vi "getObjectPrivateData.vi"(8 "error in (no error)":errorcluster, 10 "object in":refnum<class>) -> (0 "error out":errorcluster, 3 "private data":variant[](array[variant]), 5 "interitance classes":string[](array[string]), 7 "versions":T1(array[cluster]))   [LabVIEW 2020, in "JKI JSON Object Serialization.lvlib" / "OOP_Utility.lvlib" / "Reflection.lvclass"]
doc: "This VI returns the class names, and private data values for the class hierarchy (top to bottom) of the input object. \n\nGCraftsman JSON Object Serialization Toolkit\nwww.GCraftsman.com\nCopyright (c) 2017, GCraftsman"
uses:
  Reflection.lvclass
  reflectionPoolAction.ctl
  Reflection.lvclass/Reflection.ctl
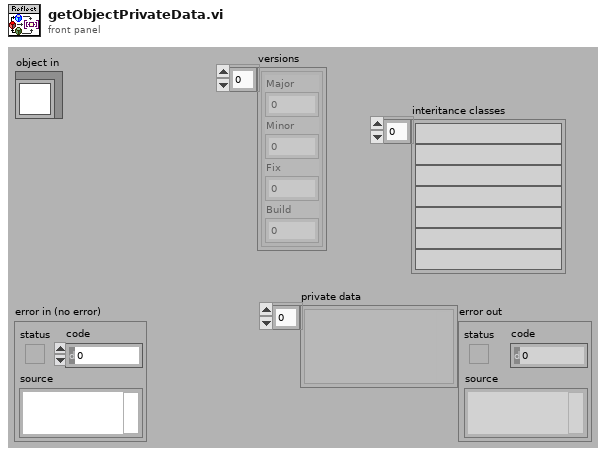
[diagram p1: front panel]
types:
  T1 = cluster{"Major":u16, "Minor":u16, "Fix":u16, "Build":u16}[]
  T2 = typedef "JKI JSON Object Serialization.lvlib/OOP_Utility.lvlib/Reflection.lvclass/reflectionPoolAction.ctl" = enum16{"<select>", "getPrivateData", "getClassHierarchy", "getClassVersions", "getAllClasses"}
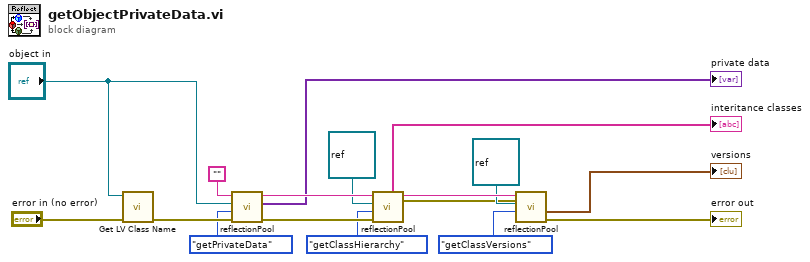
[diagram p0: block diagram]
diagram:
  n1 = call <vilib>:"Get LV Class Name.vi"("error in (no error)"="error in (no error)", "object"="object in") -> ("error out"=w16:errorcluster)  [unwired: 8 in, 1 out]
  n2 = call "reflectionPool.vi"("error in (no error)"=w16, "action"=reflectionPoolAction."getPrivateData", "object"="object in", "class name"="") -> ("error out"=w17:errorcluster, "class private data"=→"private data":variant[], "class name out"=w11:string)  [unwired: 2 in, 3 out]
  n3 = call "reflectionPool.vi"("error in (no error)"=w17, "action"=reflectionPoolAction."getClassHierarchy", "object"=refnum<class> refnum, "class name"=w11) -> ("error out"=w4:errorcluster, "class name out"=w7:string, "class hierarchy"=→"interitance classes":string[])  [unwired: 2 in, 3 out]
  n4 = call "reflectionPool.vi"("error in (no error)"=w4, "action"=reflectionPoolAction."getClassVersions", "object"=refnum<class> refnum, "class name"=w7) -> ("error out"=→"error out":errorcluster, "class version numbers"=→"versions":T1)  [unwired: 2 in, 4 out]
